vi "Write Elevator Location.vi"(8 "error in (no error)":errorcluster, 10 "Elevator Location":T1, 11 "Sim Display Console Actor in":refnum<class "Sim Display Console Actor.lvclass">) -> (0 "error out":errorcluster, 3 "Sim Display Console Actor out":refnum<class "Sim Display Console Actor.lvclass">)   [LabVIEW 2019, in "Sim Display Console Actor.lvlib" / "Sim Display Console Actor.lvclass"]
uses:
  Sim Display Console Actor.lvclass
  Floors -Enum.ctl
  Sim Display Console Actor.lvclass/Sim Display Console Actor.ctl
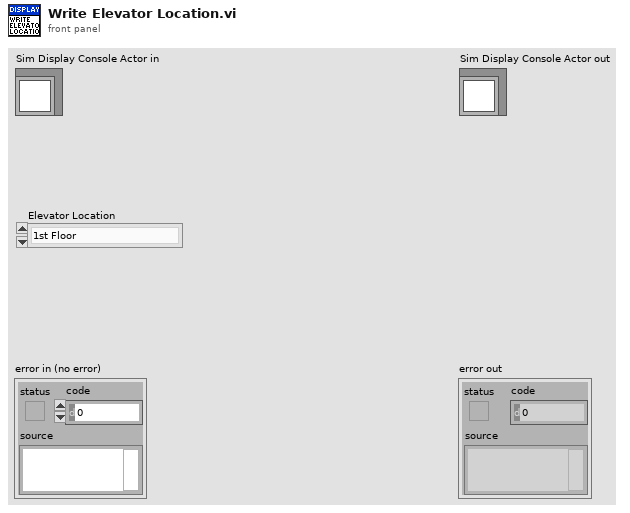
[diagram p1: front panel]
types:
  T1 = typedef "Sim Display Console Actor.lvlib/Sim Display Console Actor.lvclass/Floors -Enum.ctl" = enum16{"1st Floor", "2nd Floor", "3rd Floor", "4th Floor"}
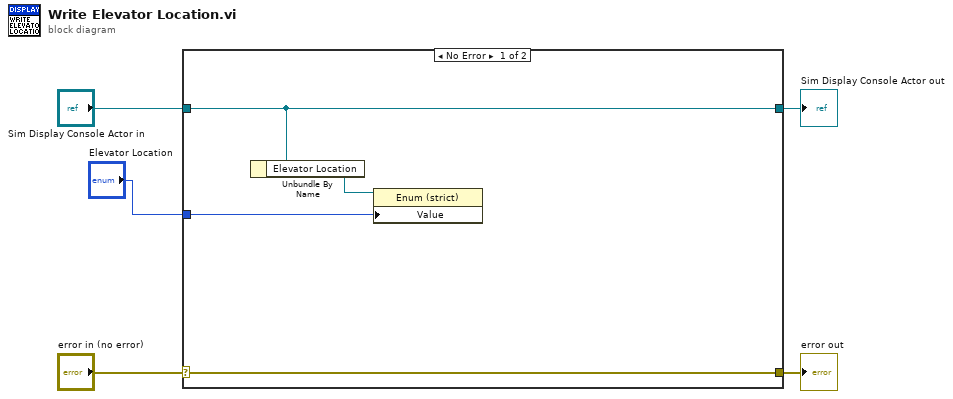
[diagram p0: block diagram]
diagram:
  n1 = case shown="No Error" "error in (no error)" {
    selector: "error in (no error)" -> [w9 w11]
    tunnel: [w9 w11] -> w4
    tunnel: [w8 w10] -> w2
    tunnel: "Sim Display Console Actor in" -> [w8 w10]
    tunnel: "Elevator Location" -> [w6 _]
    frame No Error {
      n2 = Unbundle By Name(w8) -> ("Elevator Location"=w7:refnum<vi>)
      n3 = property class="Enum (strict)"(reference=w7, "Value"=w6) -> ()  [unwired: 1 in, 2 out]
    }
    frame Error {
    }
  }
  "error out" <- w4
  "Sim Display Console Actor out" <- w2
